vi "Find The Most File 2012 NIVerified.vi"(6 "pattern":string, 8 "error in":errorcluster, 10 "file(T)/folder(F)":bool=TRUE, 11 "Folder Path In":path) -> (0 "error out":errorcluster, 3 "File Path Out":path=path "E:/20250409-103904beads-cropbulkcalib")   [LabVIEW 2024]
panel:
  # "Overview: This VI takes in a listing of files from a folder path, finds out all the files in the folder, and returns the path to the most recent file.\nRequirements: LabVIEW Base Development System\nInstructions:\n1. Select folder for searching most recent file.\n2. Run VI.\n3. Observe most recent file at File Path Out indicator."
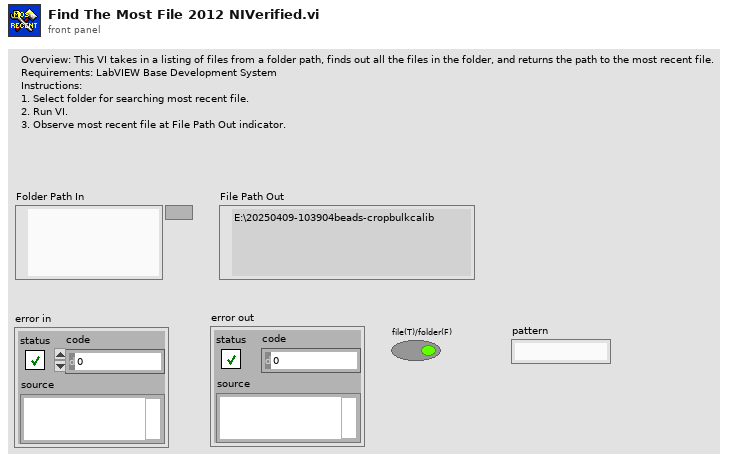
[diagram p1: front panel]
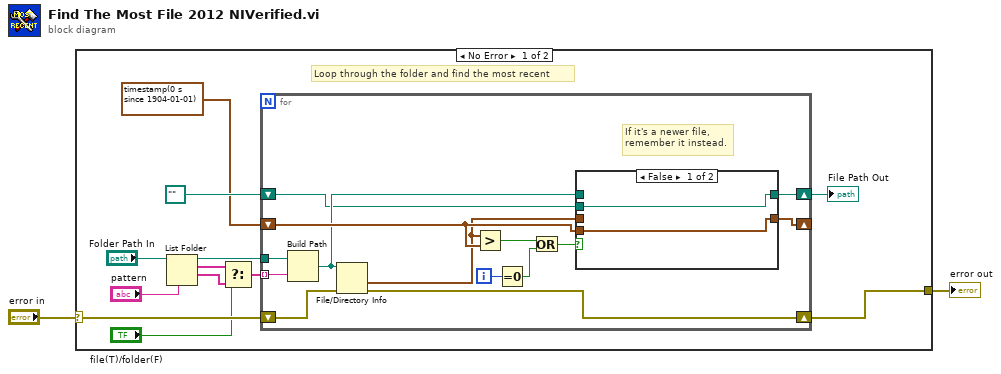
[diagram p0: block diagram]
diagram:
  n1 = case shown="No Error" "error in" {
    selector: "error in" -> [w10 w33]
    tunnel: [w14 w33] -> w2
    frame No Error {
      # "Loop through the folder and find the most recent"
      n2 = List Folder(path="Folder Path In", pattern="pattern") -> (path out=w8:path, filenames=w6:string[], folder names=w5:string[])  [unwired: 2 in, 1 out]
      n3 = Select(t=w6, s="file(T)/folder(F)", f=w5) -> (s? t:f=w7:string[])
      n4 = for {
        shift-right: [w22] -> _
        shift-left: timestamp(0 s since 1904-01-01) ("last mod 2") -> [w23]
        shift-right: [w19] -> w13
        shift-left: path "" -> [w18]
        shift-right: [w17] -> w14
        shift-left: w10 -> [w28]
        tunnel: w7 -> [w16] mode=indexing
        tunnel: w8 -> [w15]
        i -> [w24]
        # "If it's a newer file,\nremember it instead."
        n5 = Build Path(base path=w15, name or relative path=w16) -> (appended path=w20:path)
        n6 = File/Directory Info(path=w20, error in=w28) -> (last mod=w21:timestamp, error out=w17:errorcluster)  [unwired: 5 out]
        n7 = Greater?(x=w21, y=w23) -> (0:w26:bool)
        n8 = Equal To 0?(x=w24) -> (x = 0?=w25:bool)
        n9 = Or(x=w26, y=w25) -> (x .or. y?=w27:bool)
        n10 = case shown="False" w27 {
          tunnel: w23 -> [w30 _]
          tunnel: [w30 w32] -> w22
          tunnel: w21 -> [_ w32]
          tunnel: w20 -> [_ w31]
          tunnel: [w29 w31] -> w19
          tunnel: w18 -> [w29 _]
          frame False {
          }
          frame True {
          }
        }
      }
      "File Path Out" <- w13
    }
    frame Error {
      # "If there is any error, do not do anything."
    }
  }
  "error out" <- w2
